vi "Robot Global Data.vi"() -> ()   [LabVIEW 2015]
doc: "This global VI can contain as many global variables as you need. Place a control on the panel, give it a good name. To read or write to it from a VI, drag the icon to the diagram of that VI. You can also drag from the project. Click on the node to change which global you access. You shouldn't have multiple locations writing to a global or it will cause a race-condition."
uses:
  <vilib>/Rock Robotics/WPI/Camera/WPI_CameraImageSize.ctl
panel:
  in  "Turn":bool
  out "Done":bool
  in  "Shoot":bool
  in  "Turn Angle":dbl
  in  "Distance":dbl
  in  "Shoot Speed":dbl=1.0
  in  "Shoot Ball":bool
  in  "Ball Start":bool
  out "Robot Mode":i32
  in  "Auto Go":bool
  in  "Joystick Y":dbl
  in  "Joystick X":dbl
  out "ms to process":u32
  out "Detected Totes":T1(array[cluster]) {"Normalized Rect"."Numeric 5" format="%#_2g"; "Normalized Rect"."Numeric 3" format="%#_2g"; "Normalized Rect"."Numeric 2" format="%#_2g"; "Normalized Rect"."Numeric" format="%#_2g"}
  in  "image size":T2=enum."320x240"
  in  "Enable Vision":bool
  # "Autonomous Functions"
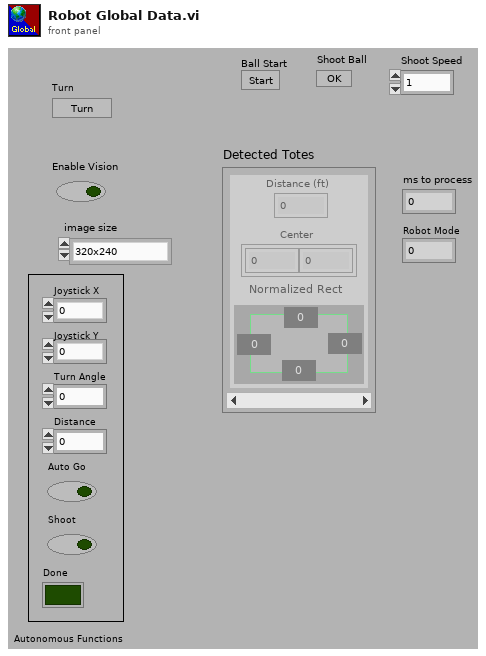
[diagram p1: front panel]
types:
  T1 = cluster{"Distance (ft)":dbl, "Center":cluster{dbl, dbl}, "Normalized Rect":cluster{"Numeric":dbl, "Numeric 2":dbl, "Numeric 3":dbl, "Numeric 5":dbl}}[]
  T2 = typedef "WPI_CameraImageSize.ctl" = enum16{"640x480", "320x240", "160x120", "Custom"}
diagram:
